vi "CRC16_Calculator.vi"(5 "ByteOrder":bool, 6 "ReverseCRC":bool, 7 "LSB First":bool, 8 "Postcond":bool, 9 "Precond":bool, 10 "Polynom":u16=4129 format="%.0x", 11 "String in":string) -> (1 "Bytes":u8[](array[numeric]) format="%.0x", 2 "Numeric":u16 format="%.0x", 3 "CRC16 out":string)   [LabVIEW 2015, in "Ion Motion Roboclaw.lvlib"]
doc: "This is a general 16 bit CRC calculation VI.\n\nThe standard inputs will calculate the CRC with the following conditions:\n\nPolynom: x^16+x^12+x^5+1\nPrecondition: 0x0000\nPostcondition: not inverting\nMost significant bit of a byte first\nCRC output not bitwise reversed\nMost significant byte first\n\nThe input \"Check this message!\" will generate an output of 0x9E8F.\n\nThe VI was started by Shane aka shoneill in the NI Developer Zone. He implemented the HW like algorithm in the inner loop. Many thanks to him.\n\nThis VI was created and tested for the Intel plattform. I'm not sure that the byte order will be correct on a Motorola plattform."
uses:
  <instrlib>/Ion Motion Roboclaw/Ion Motion Roboclaw.lvlib
panel:
  # "Input"
  # "Conditioning"
  # "Bitsequence"
  # "Output Byte Order"
  # "Output"
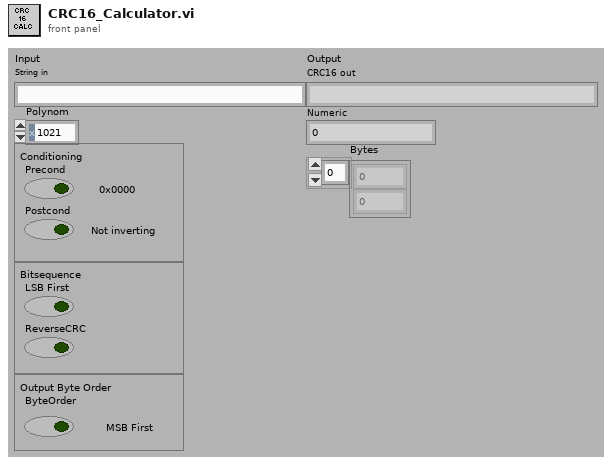
[diagram p1: front panel]
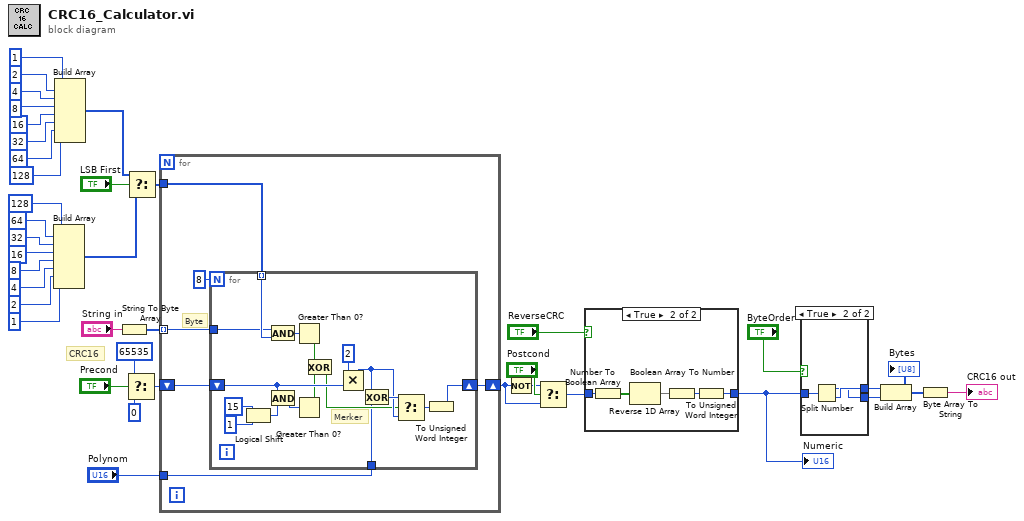
[diagram p0: block diagram]
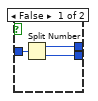
[diagram p2: hidden frame]
diagram:
  # "CRC16"
  n1 = Build Array(u8 128, u8 64, u8 32, u8 16, u8 8, u8 4, u8 2, u8 1) -> (w15:u8[])
  n2 = Build Array(u8 1, u8 2, u8 4, u8 8, u8 16, u8 32, u8 64, u8 128) -> (w14:u8[])
  n3 = String To Byte Array(string="String in") -> (unsigned byte array=w37:u8[])
  n4 = Select(t=u16 65535, s="Precond", f=u16 0) -> (s? t:f=w36:u16)
  n5 = Select(t=w14, s="LSB First", f=w15) -> (s? t:f=w17:u8[])
  n6 = for {
    shift-right: [w42] -> w11
    shift-left: w36 -> [w44]
    tunnel: w37 -> [w41] mode=indexing
    tunnel: w17 -> [w40]
    tunnel: "Polynom" -> [w39]
    # "Byte"
    n7 = for {
      N: 8 -> [_]
      shift-right: [w60] -> w42
      shift-left: w44 -> [w50]
      tunnel: w40 -> [w51] mode=indexing
      tunnel: w41 -> [w46]
      tunnel: w39 -> [w45]
      # "Merker"
      n8 = Logical Shift(y=u16 15, x=u16 1) -> (x << y=w54:u16)
      n9 = And(x=w46, y=w51) -> (x .and. y?=w58:u8)
      n10 = And(x=w50, y=w54) -> (x .and. y?=w53:u16)
      n11 = Greater Than 0?(x=w58) -> (x > 0?=w57:bool)
      n12 = Greater Than 0?(x=w53) -> (x > 0?=w48:bool)
      n13 = Exclusive Or(1:w48, 2:w57) -> (0:w47:bool)
      n14 = Multiply(x=u16 2, y=w50) -> (x*y=w52:u16)
      n15 = Exclusive Or(1:w45, 2:w52) -> (0:w61:u16)
      n16 = Select(t=w61, s=w47, f=w52) -> (s? t:f=w59:u16)
      n17 = To Unsigned Word Integer(number=w59) -> (unsigned 16bit integer=w60:u16)
    }
  }
  n18 = Not(x=w11) -> (.not. x?=w10:u16)
  n19 = Select(t=w10, s="Postcond", f=w11) -> (s? t:f=w9:u16)
  n20 = case shown="True" "ReverseCRC" {
    tunnel: w9 -> [w62 w67]
    tunnel: [w62 w63] -> w1
    frame False {
    }
    frame True {
      n21 = Number To Boolean Array(number=w67) -> (Boolean array=w66:bool[])
      n22 = Reverse 1D Array(array=w66) -> (reversed array=w65:bool[])
      n23 = Boolean Array To Number(Boolean array=w65) -> (number=w64:u32)
      n24 = To Unsigned Word Integer(number=w64) -> (unsigned 16bit integer=w63:u16)
    }
  }
  "Numeric" <- w1
  n25 = case shown="True" "ByteOrder" {
    tunnel: w1 -> [w70 w73]
    tunnel: [w69 w72] -> w2
    tunnel: [w68 w71] -> w3
    frame False {
      n26 = Split Number(x=w70) -> (hi(x)=w69:u8, lo(x)=w68:u8)
    }
    frame True {
      n27 = Split Number(x=w73) -> (hi(x)=w71:u8, lo(x)=w72:u8)
    }
  }
  n28 = Build Array(w2, w3) -> (w5:u8[])
  "Bytes" <- w5
  n29 = Byte Array To String(unsigned byte array=w5) -> (string=→"CRC16 out":string)
